vi "Align cRIO Programming Mode.vi"(5 "Password":string, 7 "User Name":string, 8 "error in (no error)":errorcluster, 9 "List of Products":string[](array[string])=["cRIO-9040", "cRIO-9041", "cRIO-9042", "cRIO-9043", "cRIO-9044", "cRIO-9045", "cRIO-9046", "cRIO-9047", "cRIO-9048", "cRIO-9049", "cRIO-9056", "cRIO-9057"], 10 "FPGAScanInterfaceMode":u16, 11 "Target (localhost)":refnum<k21>="localhost") -> (0 "error out":errorcluster, 2 "Slots Information":T1(array[cluster]) {"Programming Mode" items=["None"=0, "Real-Time CPU"=1, "Real-Time Scan Engine"=2, "LabVIEW FPGA"=4]}, 3 "Slot Programming Mode Supported?":bool)   [LabVIEW 2016, in "Scan Engine Custom Device.lvlib"]
doc: "Based on FPGAScanInterfaceMode input, this VI aligns actual Slot Programming Mode:\n- FPGAScanInterfaceMode = 0 (Use Current), we do nothing. We don't even check current settings (because, it's super slow (SystemConfiguration API)).\n- FPGAScanInterfaceMode = 1 (FPGA) or (Scan mode), we retrieves Product Name and if it's a ni-rio product, checks agains Input list whether it supports the Slot Programming Mode. Then, for detected Slots, we ensure the Slot Programming Mode value is aligned to FPGAScanInterfaceMode and change it if required."
uses:
  <vilib>/nisyscfg/Filter Mode.ctl
  <vilib>/nisyscfg/Save Changes (Hardware).vi
  <vilib>/nisyscfg/Close (Hardware).vi
  <vilib>/nisyscfg/Close (Filter).vi
  <vilib>/nisyscfg/Close (System).vi
  Scan Engine Custom Device.lvlib
  <vilib>/nisyscfg/nisyscfg.lvlib
  <resource>/objmgr/nicontrollersysapi.rc
  <resource>/objmgr/niflexriosae.rc
panel:
  # "FPGAScanInterfaceMode:\n0: Use Current\n1: FPGA\n2: Scan mode"
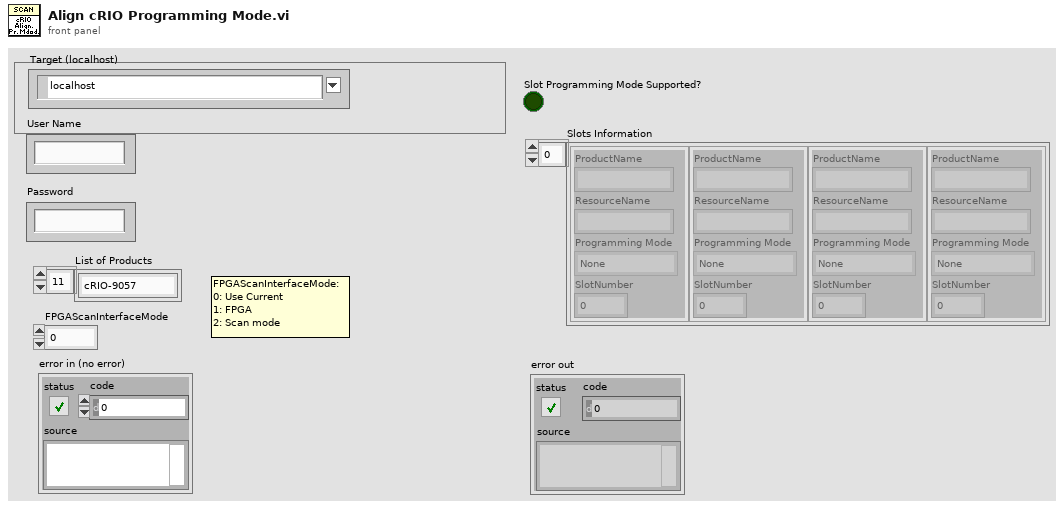
[diagram p1: front panel]
types:
  T1 = cluster{"ProductName":string, "ResourceName":string, "Programming Mode":u32, "SlotNumber":i32}[]
  T2 = cluster{"ProductName":string, "ResourceName":string, "Programming Mode":u32, "SlotNumber":i32}
  T3 = typedef "nisyscfg.lvlib/Filter Mode.ctl" = i32
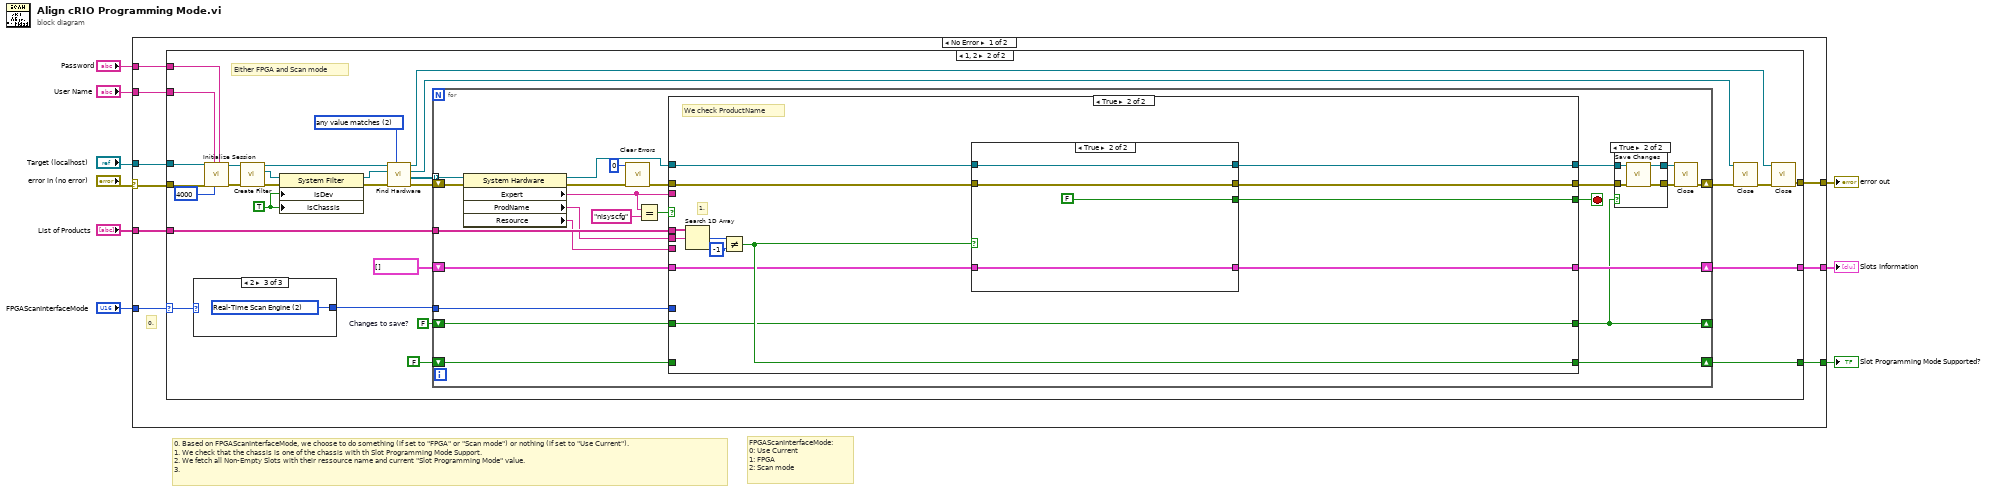
[diagram p0: block diagram]
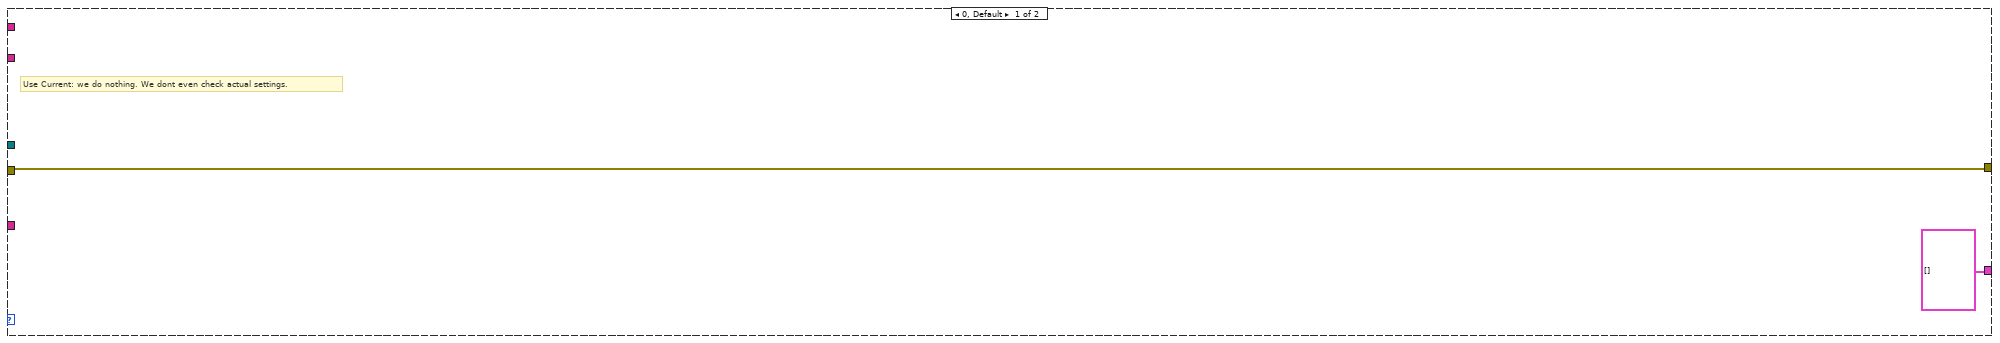
[diagram p2: hidden frame]
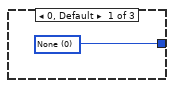
[diagram p3: hidden frame]
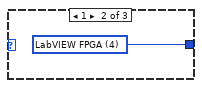
[diagram p4: hidden frame]
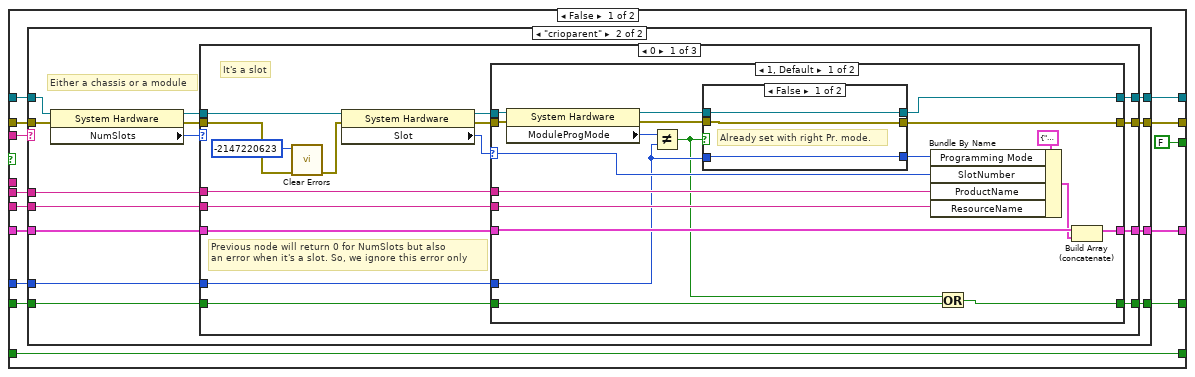
[diagram p6: hidden frame]
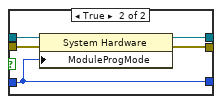
[diagram p8: hidden frame]
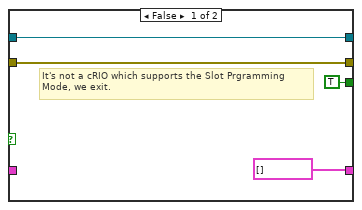
[diagram p12: hidden frame]
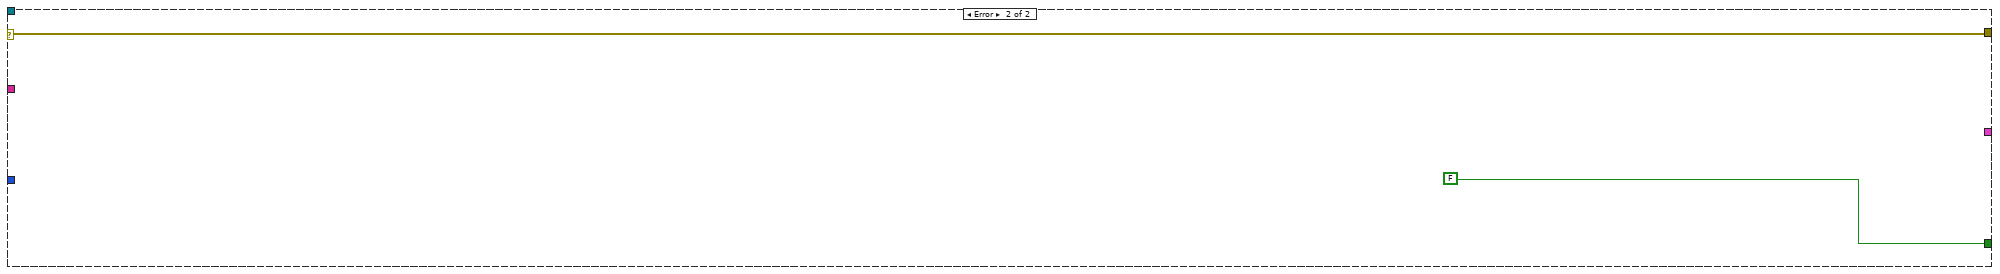
[diagram p13: hidden frame]
diagram:
  # "FPGAScanInterfaceMode:\n0: Use Current\n1: FPGA\n2: Scan mode"
  # "0. Based on FPGAScanInterfaceMode, we choose to do something (if set to \"FPGA\" or \"Scan mode\") or nothing (if set to \"Use Current\"). \n1. We check that the chassis is one of the chassis with th Slot Programming Mode Support.\n2. We fetch all Non-Empty Slots with their ressource name and current \"Slot Programming Mode\" value.\n3."
  n1 = case shown="No Error" "error in (no error)" {
    selector: "error in (no error)" -> [w12 w193]
    tunnel: "Target (localhost)" -> [w18 _]
    tunnel: "User Name" -> [w17 _]
    tunnel: "Password" -> [w16 _]
    tunnel: "List of Products" -> [w15 _]
    tunnel: [w14 FALSE] -> w5
    tunnel: [w13 w193] -> w4
    tunnel: [w11 _] -> w2
    tunnel: "FPGAScanInterfaceMode" -> [w10 _]
    frame No Error {
      # "0."
      n2 = case shown="1, 2" w10 {
        selector: w10 -> [_ w23]
        tunnel: w18 -> [_ w35]
        tunnel: w17 -> [_ w34]
        tunnel: w16 -> [_ w33]
        tunnel: w15 -> [_ w30]
        tunnel: [_ w29] -> w14
        tunnel: [w20 w28] -> w13
        tunnel: w12 -> [w20 w27]
        tunnel: [T1 [] w24] -> w11
        frame 0, Default {
          # "Use Current: we do nothing. We dont even check actual settings."
        }
        frame 1, 2 {
          w21 = FALSE  # Changes to save?
          w40 = T3 2 items=["all values match"=1, "any value matches"=2, "values do not match"=3, "all properties exist"=4] ("filter mode (all values match)")
          w32 = TRUE ("Is Chassis")
          # "Either FPGA and Scan mode"
          n3 = case shown="2" w23 {
            tunnel: [w50 w51 w52] -> w22
            frame 0, Default {
              w50 = u32 0 items=["None"=0, "Real-Time CPU"=1, "Real-Time Scan Engine"=2, "LabVIEW FPGA"=4] ("Programming Mode")
            }
            frame 1 {
              w51 = u32 4 items=["None"=0, "Real-Time CPU"=1, "Real-Time Scan Engine"=2, "LabVIEW FPGA"=4] ("Programming Mode")
            }
            frame 2 {
              w52 = u32 2 items=["None"=0, "Real-Time CPU"=1, "Real-Time Scan Engine"=2, "LabVIEW FPGA"=4] ("Programming Mode")
            }
          }
          n4 = call <vilib>:"Initialize Session.vi"("Password"=w33, "Connect Timeout (4000 ms)"=u32 4000, "User Name"=w34, "error in (no error)"=w27, "Target (localhost)"=w35) -> ("error out"=w42:errorcluster, "Session out"=w45:refnum<k21>)  [unwired: 5 in]
          n5 = call <vilib>:"Create Filter.vi"("error in (no error)"=w42, "Session in"=w45) -> ("error out"=w47:errorcluster, "Filter out"=w46:refnum<k20>, "Session out"=w44:refnum<k21>)  [unwired: 7 in]
          n6 = property class="System Filter"(reference=w46, error in=w47, "IsDev"=w32, "IsChassis"=w32) -> (reference out=w41:refnum<k20>, error out=w43:errorcluster)
          n7 = call <vilib>:"Find Hardware.vi"("Filter Mode (all values match)"=w40, "error in (no error)"=w43, "Filter in"=w41, "Session in"=w44) -> ("error out"=w36:errorcluster, "Resources out"=w49:refnum<k20>[], "Filter out"=w38:refnum<k20>, "Session out"=w48:refnum<k21>)  [unwired: 4 out]
          n8 = for {
            tunnel: w49 -> [w76] mode=indexing
            shift-right: [w77] -> w37
            shift-left: w36 -> [w74]
            tunnel: w30 -> [w71]
            shift-right: [w70] -> w29
            shift-left: FALSE -> [w66]
            shift-right: [w62] -> w24
            shift-left: T1 [] -> [w63]
            tunnel: w22 -> [w59]
            shift-right: [w53] -> _
            shift-left: w21 -> [w58]
            stop <- w65 stop-if-true
            n9 = property class="System Hardware"(reference=w76, error in=w74) -> (reference out=w68:refnum<k20>, error out=w75:errorcluster, "Expert"=w61:string, "ProdName"=w69:string, "Resource"=w64:string)
            n10 = call <vilib>:"Clear Errors.vi"("error in (no error)"=w75, "specific error code to clear (0: all)"=0) -> ("error out"=w67:errorcluster)  [unwired: 4 in, 1 out]
            n11 = Equal?(x=w61, y="nisyscfg") -> (x = y?=w72:bool)
            n12 = case shown="True" w72 {
              tunnel: w69 -> [w88 w182]
              tunnel: w71 -> [_ w183]
              tunnel: [w97 w179] -> w70
              tunnel: w68 -> [w93 w177]
              tunnel: w67 -> [w95 w178]
              tunnel: [w94 w176] -> w56
              tunnel: [w92 w175] -> w57
              tunnel: w66 -> [w97 _]
              tunnel: [FALSE w174] -> w65
              tunnel: w64 -> [w91 _]
              tunnel: w63 -> [w90 w173]
              tunnel: [w89 w172] -> w62
              tunnel: w61 -> [w87 _]
              tunnel: w59 -> [w86 _]
              tunnel: w58 -> [w85 w171]
              tunnel: [w84 w171] -> w53
              frame False {
                n13 = case shown="\"crioparent\"" w87 {
                  tunnel: w95 -> [w101 w114]
                  tunnel: [w101 w107] -> w94
                  tunnel: w93 -> [w100 w115]
                  tunnel: [w100 w108] -> w92
                  tunnel: w91 -> [_ w106]
                  tunnel: w90 -> [w99 w110]
                  tunnel: [w99 w109] -> w89
                  tunnel: w88 -> [_ w105]
                  tunnel: w86 -> [_ w104]
                  tunnel: w85 -> [w98 w103]
                  tunnel: [w98 w102] -> w84
                  frame Default {
                  }
                  frame "crioparent" {
                    # "Either a chassis or a module"
                    n14 = property class="System Hardware"(reference=w115, error in=w114) -> (reference out=w112:refnum<k20>, error out=w111:errorcluster, "NumSlots"=w113:i32)
                    n15 = case shown="0" w113 {
                      tunnel: w112 -> [w125 w166 w169]
                      tunnel: w111 -> [w120 w165 w168]
                      tunnel: w110 -> [w129 w164 w170]
                      tunnel: [w128 w164 w170] -> w109
                      tunnel: [w131 w166 w169] -> w108
                      tunnel: [w130 w165 w168] -> w107
                      tunnel: w106 -> [w127 _ _]
                      tunnel: w105 -> [w126 _ _]
                      tunnel: w104 -> [w121 _ _]
                      tunnel: w103 -> [w117 w163 w167]
                      tunnel: [w116 w163 w167] -> w102
                      frame 0 {
                        # "Previous node will return 0 for NumSlots but also\nan error when it's a slot. So, we ignore this error only"
                        # "It's a slot"
                        n16 = call <vilib>:"Clear Errors.vi"("error in (no error)"=w120, "specific error code to clear (0: all)"=-2147220623) -> ("error out"=w119:errorcluster)  [unwired: 4 in, 1 out]
                        n17 = property class="System Hardware"(reference=w125, error in=w119) -> (reference out=w123:refnum<k20>, error out=w122:errorcluster, "Slot"=w124:i32)
                        n18 = case shown="1, Default" w124 {
                          selector: w124 -> [w145 _]
                          tunnel: w123 -> [w150 w162]
                          tunnel: [w138 w162] -> w131
                          tunnel: w122 -> [w149 w161]
                          tunnel: [w136 w161] -> w130
                          tunnel: w129 -> [w148 w160]
                          tunnel: [w147 w160] -> w128
                          tunnel: w127 -> [w142 _]
                          tunnel: w126 -> [w143 _]
                          tunnel: w121 -> [w137 _]
                          tunnel: w117 -> [w133 w159]
                          tunnel: [w132 w159] -> w116
                          frame 1, Default {
                            n19 = property class="System Hardware"(reference=w150, error in=w149) -> (reference out=w140:refnum<k20>, error out=w139:errorcluster, "ModuleProgMode"=w141:u32)
                            n20 = Not Equal?(x=w141, y=w137) -> (x != y?=w134:bool)
                            n21 = case shown="False" w134 {
                              tunnel: w140 -> [w153 w158]
                              tunnel: w139 -> [w152 w156]
                              tunnel: [w153 w157] -> w138
                              tunnel: w137 -> [w151 w154]
                              tunnel: [w152 w155] -> w136
                              tunnel: [w151 w154] -> w135
                              frame False {
                                # "Already set with right Pr. mode."
                              }
                              frame True {
                                n22 = property class="System Hardware"(reference=w158, error in=w156, "ModuleProgMode"=w154) -> (reference out=w157:refnum<k20>, error out=w155:errorcluster)
                              }
                            }
                            n23 = Bundle By Name(cluster=T2 {"ProductName"="", "ResourceName"="", "Programming Mode"=0, "SlotNumber"=0}, "Programming Mode"=w135, "SlotNumber"=w145, "ProductName"=w143, "ResourceName"=w142) -> (w144:T2)
                            n24 = Or(x=w134, y=w133) -> (x .or. y?=w132:bool)
                            n25 = Build Array (concatenate)(w148, w144) -> (w147:T1)
                          }
                          frame -1, 0 {
                          }
                        }
                      }
                      frame -1, Default {
                        # "This case should\nnever happen."
                      }
                      frame 4, 8 {
                        # "It's a chassis"
                      }
                    }
                  }
                }
              }
              frame True {
                # "1."
                # "We check ProductName"
                n26 = Search 1D Array(1D array=w183, element=w182) -> (index of element=w181:i32)  [unwired: 1 in]
                n27 = Not Equal?(x=w181, y=-1) -> (x != y?=w179:bool)
                n28 = case shown="True" w179 {
                  tunnel: w178 -> [w186 w189]
                  tunnel: w177 -> [w187 w190]
                  tunnel: [w186 w189] -> w176
                  tunnel: [w187 w190] -> w175
                  tunnel: [TRUE FALSE] -> w174
                  tunnel: w173 -> [_ w188]
                  tunnel: [T1 [] w188] -> w172
                  frame False {
                    # "It's not a cRIO which supports the Slot Prgramming\nMode, we exit."
                  }
                  frame True {
                  }
                }
              }
            }
            n29 = case shown="True" w53 {
              tunnel: w57 -> [w79 w83]
              tunnel: w56 -> [w78 w82]
              tunnel: [w78 w81] -> w55
              tunnel: [w79 w80] -> w54
              frame False {
              }
              frame True {
                n30 = call-poly <vilib>:"Save Changes.vi"("error in (no error)"=w82, "Resource in"=w83) -> ("error out"=w81:errorcluster, "Resource out"=w80:refnum<k20>)  [unwired: 6 in, 2 out]
              }
            }
            n31 = call-poly <vilib>:"Close.vi"("error in (no error)"=w55, "Resource in"=w54) -> ("error out"=w77:errorcluster)  [unwired: 9 in]
          }
          n32 = call-poly <vilib>:"Close.vi"("error in (no error)"=w37, "Filter in"=w38) -> ("error out"=w39:errorcluster)  [unwired: 9 in]
          n33 = call-poly <vilib>:"Close.vi"("error in (no error)"=w39, "Session in"=w48) -> ("error out"=w28:errorcluster)  [unwired: 9 in]
        }
      }
    }
    frame Error {
    }
  }
  "Slot Programming Mode Supported?" <- w5
  "error out" <- w4
  "Slots Information" <- w2
